vi "复杂计算器.vi"() -> ()   [LabVIEW 2018]
panel:
  in  "等于":bool
  in  "清除":bool
  in  "除":bool
  in  "小数点":bool
  in  "0":bool
  in  "正负号":bool
  in  "乘":bool
  in  "9":bool
  in  "8":bool
  in  "7":bool
  in  "减":bool
  in  "6":bool
  in  "5":bool
  in  "4":bool
  in  "加":bool
  in  "3":bool
  in  "2":bool
  in  "1":bool
  out "结果":string
  out "输入1":string
  out "输入2":string
  out "输入临时值":string
  out "操作临时值":string
  out "显示过程":string
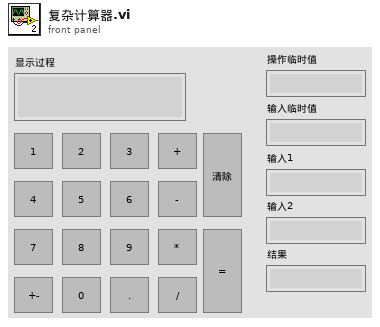
[diagram p1: front panel]
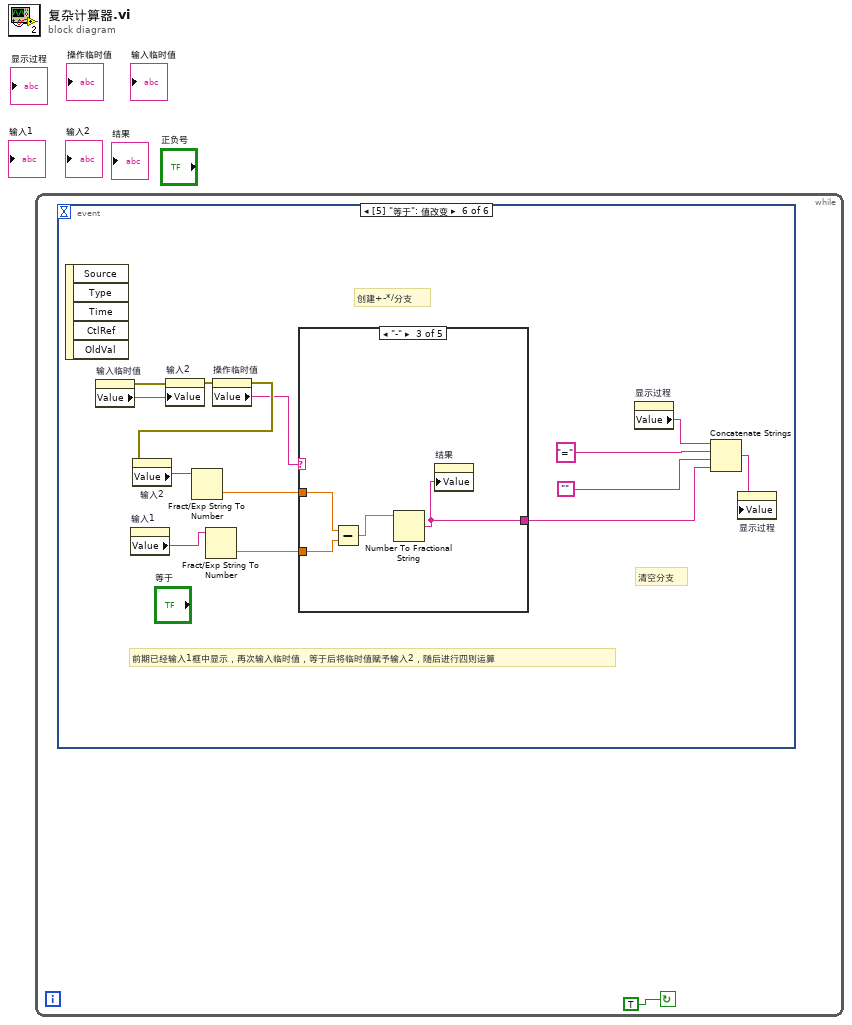
[diagram p0: block diagram]
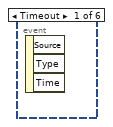
[diagram p2: hidden frame]
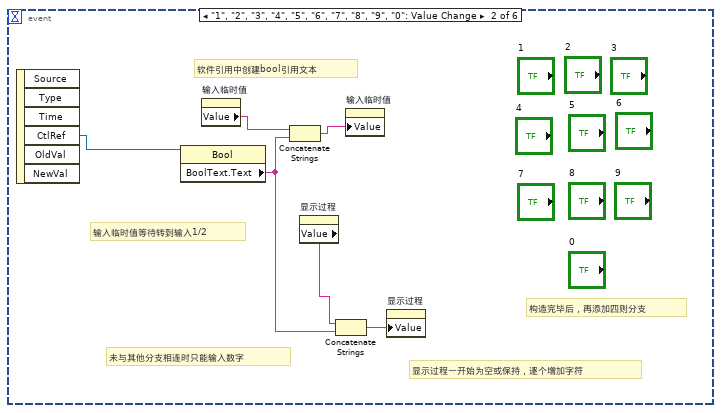
[diagram p3: hidden frame]
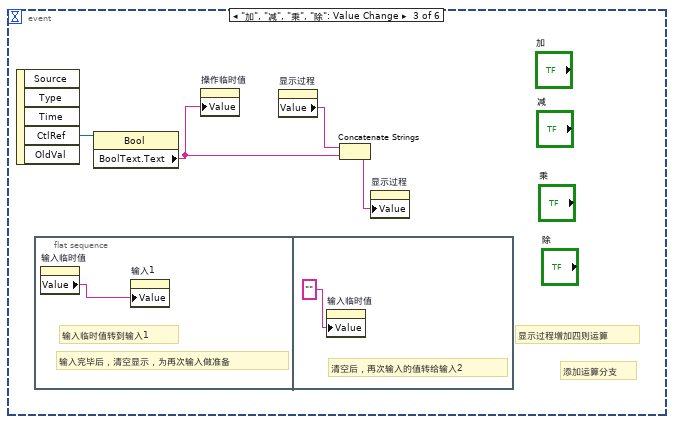
[diagram p4: hidden frame]
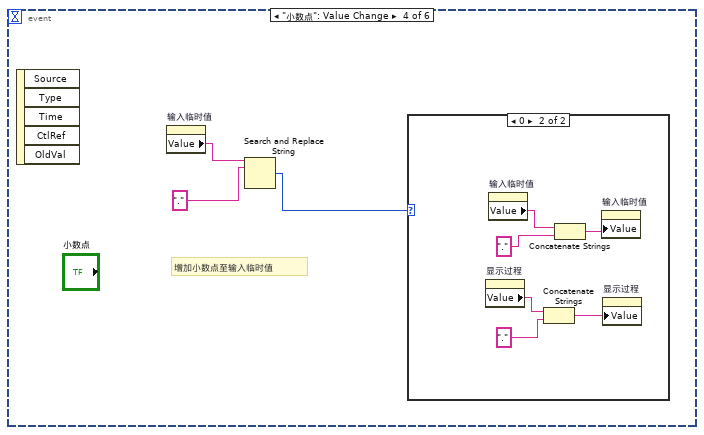
[diagram p5: hidden frame]
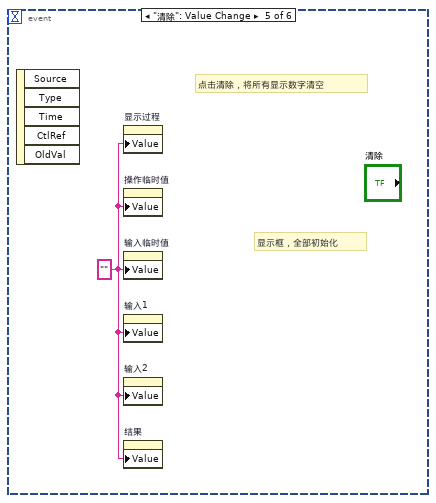
[diagram p7: hidden frame]
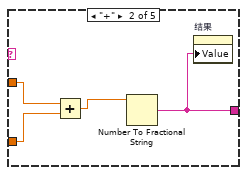
[diagram p9: hidden frame]
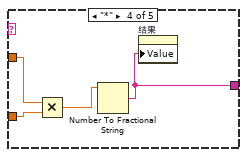
[diagram p10: hidden frame]
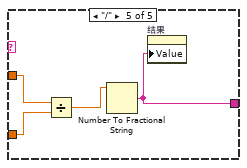
[diagram p11: hidden frame]
diagram:
  n1 = while {
    stop <- TRUE continue-if-true
    n2 = event shown="[5] \"等于\": 值改变" {
      selector: _ -> [_ _ _ _ _ _]
      dyn-events: _ -> [_ _ _ _ _ _]
      timeout: _ -> [_ _ _ _ _ _]
      event Timeout {
        n3 = event-data() -> ()  [unwired: 1 in, 3 out]
      }
      event "1", "2", "3", "4", "5", "6", "7", "8", "9", "0": Value Change {
        # "构造完毕后，再添加四则分支"
        # "输入临时值等待转到输入1/2"
        # "显示过程一开始为空或保持，逐个增加字符"
        # "未与其他分支相连时只能输入数字"
        # "软件引用中创建bool引用文本"
        n4 = event-data() -> ("CtlRef"=w2:refnum<vi>)  [unwired: 1 in, 5 out]
        n5 = property class="Bool"(reference=w2) -> ("BoolText.Text"=w3:string)  [unwired: 1 in, 2 out]
        n6 = property on="输入临时值" class="Str"() -> ("Value"=w7:string)  [unwired: 2 in, 2 out]
        n7 = Concatenate Strings(w7, w3) -> (w6:string)
        n8 = property on="显示过程" class="Str"() -> ("Value"=w5:string)  [unwired: 2 in, 2 out]
        n9 = Concatenate Strings(w5, w3) -> (w4:string)
        n10 = property on="输入临时值" class="Str"("Value"=w6) -> ()  [unwired: 2 in, 2 out]
        n11 = property on="显示过程" class="Str"("Value"=w4) -> ()  [unwired: 2 in, 2 out]
      }
      event "加", "减", "乘", "除": Value Change {
        # "添加运算分支"
        # "显示过程增加四则运算"
        n12 = event-data() -> ("CtlRef"=w11:refnum<vi>)  [unwired: 1 in, 4 out]
        n13 = flat-sequence {
          frame #0 {
            # "输入临时值转到输入1"
            # "输入完毕后，清空显示，为再次输入做准备"
            n14 = property on="输入临时值" class="Str"() -> ("Value"=w12:string)  [unwired: 2 in, 2 out]
            n15 = property on="输入1" class="Str"("Value"=w12) -> ()  [unwired: 2 in, 2 out]
          }
          frame #1 {
            # "清空后，再次输入的值转给输入2"
            n16 = property on="输入临时值" class="Str"("Value"="") -> ()  [unwired: 2 in, 2 out]
          }
        }
        n17 = property class="Bool"(reference=w11) -> ("BoolText.Text"=w9:string)  [unwired: 1 in, 2 out]
        n18 = property on="操作临时值" class="Str"("Value"=w9) -> ()  [unwired: 2 in, 2 out]
        n19 = property on="显示过程" class="Str"() -> ("Value"=w10:string)  [unwired: 2 in, 2 out]
        n20 = Concatenate Strings(w10, w9) -> (w8:string)
        n21 = property on="显示过程" class="Str"("Value"=w8) -> ()  [unwired: 2 in, 2 out]
      }
      event "小数点": Value Change {
        # "增加小数点至输入临时值"
        n22 = event-data() -> ()  [unwired: 1 in, 5 out]
        n23 = property on="输入临时值" class="Str"() -> ("Value"=w16:string)  [unwired: 2 in, 2 out]
        n24 = Search and Replace String(input string=w16, search string=".") -> (number of replacements=w14:i32)  [unwired: 6 in, 3 out]
        n25 = case shown="0" w14 {
          frame 1, Default {
          }
          frame 0 {
            n26 = property on="显示过程" class="Str"() -> ("Value"=w20:string)  [unwired: 2 in, 2 out]
            n27 = property on="输入临时值" class="Str"() -> ("Value"=w22:string)  [unwired: 2 in, 2 out]
            n28 = Concatenate Strings(w20, ".") -> (w17:string)
            n29 = Concatenate Strings(w22, ".") -> (w18:string)
            n30 = property on="输入临时值" class="Str"("Value"=w18) -> ()  [unwired: 2 in, 2 out]
            n31 = property on="显示过程" class="Str"("Value"=w17) -> ()  [unwired: 2 in, 2 out]
          }
        }
      }
      event "清除": Value Change {
        w23 = ""
        # "显示框，全部初始化"
        # "点击清除，将所有显示数字清空"
        n32 = event-data() -> ()  [unwired: 1 in, 5 out]
        n33 = property on="显示过程" class="Str"("Value"=w23) -> ()  [unwired: 2 in, 2 out]
        n34 = property on="操作临时值" class="Str"("Value"=w23) -> ()  [unwired: 2 in, 2 out]
        n35 = property on="输入临时值" class="Str"("Value"=w23) -> ()  [unwired: 2 in, 2 out]
        n36 = property on="输入1" class="Str"("Value"=w23) -> ()  [unwired: 2 in, 2 out]
        n37 = property on="输入2" class="Str"("Value"=w23) -> ()  [unwired: 2 in, 2 out]
        n38 = property on="结果" class="Str"("Value"=w23) -> ()  [unwired: 2 in, 2 out]
      }
      event "等于": Value Change {
        # "清空分支"
        # "前期已经输入1框中显示，再次输入临时值，等于后将临时值赋予输入2，随后进行四则运算"
        # "创建+-*/分支"
        n39 = event-data() -> ()  [unwired: 1 in, 5 out]
        n40 = property on="输入临时值" class="Str"() -> (error out=w36:errorcluster, "Value"=w37:string)  [unwired: 2 in, 1 out]
        n41 = property on="输入1" class="Str"() -> ("Value"=w34:string)  [unwired: 2 in, 2 out]
        n42 = property on="输入2" class="Str"(error in=w36, "Value"=w37) -> (error out=w35:errorcluster)  [unwired: 1 in, 1 out]
        n43 = Fract/Exp String To Number(string=w34) -> (number=w24:dbl)  [unwired: 3 in, 1 out]
        n44 = property on="操作临时值" class="Str"(error in=w35) -> (error out=w33:errorcluster, "Value"=w30:string)  [unwired: 1 in, 1 out]
        n45 = property on="输入2" class="Str"(error in=w33) -> ("Value"=w32:string)  [unwired: 1 in, 2 out]
        n46 = Fract/Exp String To Number(string=w32) -> (number=w31:dbl)  [unwired: 3 in, 1 out]
        n47 = case shown="\"-\"" w30 {
          tunnel: w31 -> [_ w41 w45 w49 w53]
          tunnel: w24 -> [_ w40 w44 w48 w52]
          tunnel: [_ w38 w42 w46 w50] -> w29
          frame "假", Default {
          }
          frame "+" {
            n48 = Add(x=w41, y=w40) -> (x+y=w39:dbl)
            n49 = Number To Fractional String(number=w39) -> (F-format string=w38:string)  [unwired: 3 in]
            n50 = property on="结果" class="Str"("Value"=w38) -> ()  [unwired: 2 in, 2 out]
          }
          frame "-" {
            n51 = Subtract(x=w45, y=w44) -> (x-y=w43:dbl)
            n52 = Number To Fractional String(number=w43) -> (F-format string=w42:string)  [unwired: 3 in]
            n53 = property on="结果" class="Str"("Value"=w42) -> ()  [unwired: 2 in, 2 out]
          }
          frame "*" {
            n54 = Multiply(x=w49, y=w48) -> (x*y=w47:dbl)
            n55 = Number To Fractional String(number=w47) -> (F-format string=w46:string)  [unwired: 3 in]
            n56 = property on="结果" class="Str"("Value"=w46) -> ()  [unwired: 2 in, 2 out]
          }
          frame "/" {
            n57 = Divide(x=w53, y=w52) -> (x/y=w51:dbl)
            n58 = Number To Fractional String(number=w51) -> (F-format string=w50:string)  [unwired: 3 in]
            n59 = property on="结果" class="Str"("Value"=w50) -> ()  [unwired: 2 in, 2 out]
          }
        }
        n60 = property on="显示过程" class="Str"() -> ("Value"=w26:string)  [unwired: 2 in, 2 out]
        n61 = Concatenate Strings(w26, "=", "", w29) -> (w25:string)
        n62 = property on="显示过程" class="Str"("Value"=w25) -> ()  [unwired: 2 in, 2 out]
      }
    }
  }
